vi "IDN.vi"(4 "error in":errorcluster, 6 "Address":dbl) -> (0 "error out":errorcluster, 1 "ID:":string)   [LabVIEW 2015]
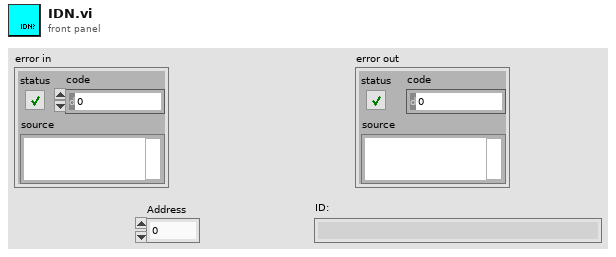
[diagram p1: front panel]
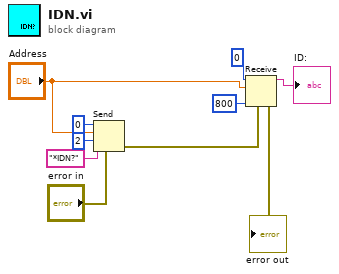
[diagram p0: block diagram]
diagram:
  n1 = Send(0:0 ("bus"), 2:"Address", 3:i16 2 ("mode"), 4:"error in", 5:"*IDN?" ("data string")) -> (8:w4:errorcluster)  [unwired: 2 out]
  n2 = Receive(4:w4, 6:800 ("count"), 8:"Address", 9:0 ("bus")) -> (0:→"error out":errorcluster, 3:→"ID:":string)  [unwired: 1 in, 2 out]
